vi "Recording Path.vi"(8 "error in (no error)":errorcluster, 11 "AODAcq in":refnum<class "AODAcq.lvclass">) -> (0 "error out":errorcluster, 2 "FilePath":path, 3 "AODAcq out":refnum<class "AODAcq.lvclass">)   [LabVIEW 2014, in "AODAcq.lvclass"]
uses:
  AODAcq.lvclass
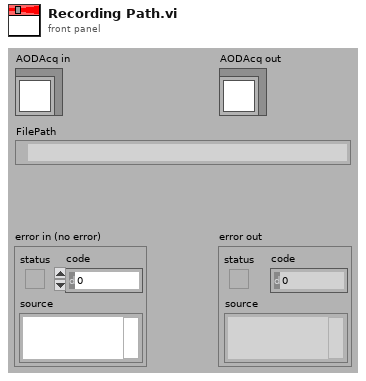
[diagram p1: front panel]
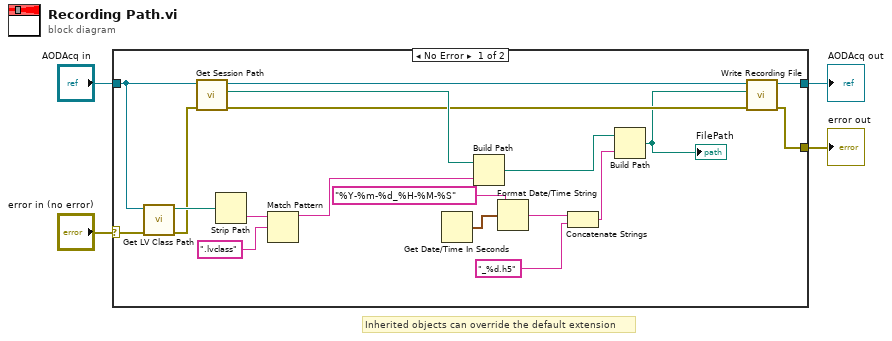
[diagram p0: block diagram]
diagram:
  # "Inherited objects can override the default extension"
  n1 = case shown="No Error" "error in (no error)" {
    selector: "error in (no error)" -> [w15 w25]
    tunnel: [w17 w25] -> w2
    tunnel: [w18 w24] -> w1
    tunnel: "AODAcq in" -> [w14 w24]
    frame No Error {
      n2 = call <vilib>:"Get LV Class Path.vi"("error in (no error)"=w15, "object"=w14) -> ("error out"=w16:errorcluster, "class path"=w21:path)  [unwired: 8 in]
      n3 = call-dynamic "Get Session Path.vi"("error in (no error)"=w16, "AcquistionObject in"=w14) -> ("error out"=w8:errorcluster, "Path"=w19:path, "AcquistionObject out"=w13:refnum<class "AODAcq.lvclass">)  [unwired: 7 in]
      n4 = Strip Path(path=w21) -> (name=w11:string)  [unwired: 1 out]
      n5 = Match Pattern(string=w11, regular expression=".lvclass") -> (before substring=w7:string)  [unwired: 1 in, 3 out]
      n6 = Get Date/Time In Seconds() -> (seconds since 1Jan1904=w22:timestamp)
      n7 = Build Path(base path=w19, name or relative path=w7) -> (appended path=w9:path)
      n8 = Format Date/Time String(time format string (%c)="%Y-%m-%d_%H-%M-%S", seconds (now)=w22) -> (date/time string=w6:string)  [unwired: 1 out]
      n9 = Concatenate Strings(w6, "_%d.h5" ("string")) -> (w20:string)
      n10 = Build Path(base path=w9, name or relative path=w20) -> (appended path=w5:path)
      "FilePath" <- w5
      n11 = call-dynamic "Write Recording File.vi"("error in (no error)"=w8, "Recording File"=w5, "AcquistionObject in"=w13) -> ("error out"=w17:errorcluster, "AcquistionObject out"=w18:refnum<class "AODAcq.lvclass">)  [unwired: 7 in]
    }
    frame Error {
    }
  }
  "error out" <- w2
  "AODAcq out" <- w1
